vi "SQLDrivers.vi"(4 "error in (no error)":errorcluster, 7 "EnvHandle":i32) -> (0 "error out":errorcluster, 1 "DriverAttributes":string, 2 "DriverDescription":string, 3 "dup EnvHandle":i32)   [LabVIEW 2011]
doc: "Se connecte auprès de la base spécifiée. S'identifie par le nom d'utilisateur et le mot de passe associé"
uses:
  Odbc32.dll
panel:
  out "Overflow 2":i16
  out "Overflow 1":i16
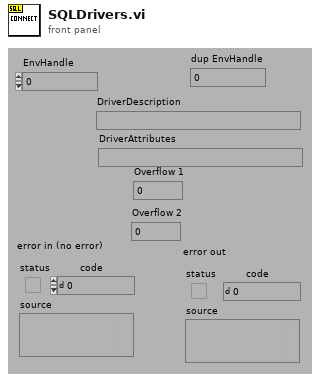
[diagram p1: front panel]
types:
  T1 = enum16{"NOPE", "SQL_HANDLE_ENV", "SQL_HANDLE_DBC", "SQL_HANDLE_STMT", "SQL_HANDLE_DESC"}
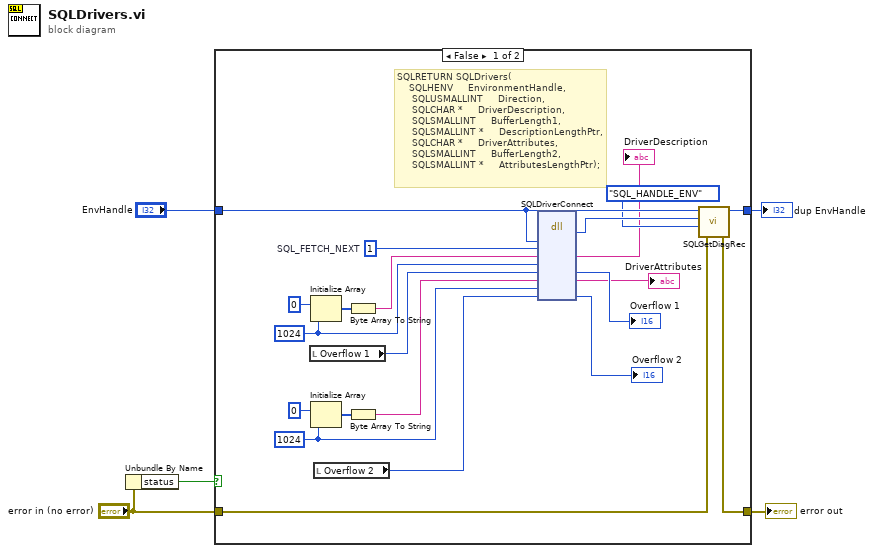
[diagram p0: block diagram]
diagram:
  n1 = Unbundle By Name("error in (no error)") -> ("status"=w4:bool)
  n2 = case shown="False" w4 {
    tunnel: "EnvHandle" -> [w26 w28]
    tunnel: "error in (no error)" -> [w24 w27]
    tunnel: [w23 w27] -> w3
    tunnel: [w25 w28] -> w2
    frame False {
      w9 = i16 1024 ("dimension size")
      w18 = u16 1  # SQL_FETCH_NEXT
      w16 = i16 1024 ("dimension size")
      # "SQLRETURN SQLDrivers(\n    SQLHENV     EnvironmentHandle,\n     SQLUSMALLINT     Direction,\n     SQLCHAR *     DriverDescription,\n     SQLSMALLINT     BufferLength1,\n     SQLSMALLINT *     DescriptionLengthPtr,\n     SQLCHAR *     DriverAttributes,\n     SQLSMALLINT     BufferLength2,\n     SQLSMALLINT *     AttributesLengthPtr);"
      n3 = local read "Overflow 1"() -> (w13:i16)
      n4 = Initialize Array(u8 0, w16) -> (w19:u8[])
      n5 = Initialize Array(u8 0, w9) -> (w12:u8[])
      n6 = local read "Overflow 2"() -> (w8:i16)
      n7 = Byte Array To String(unsigned byte array=w19) -> (string=w17:string)
      n8 = Byte Array To String(unsigned byte array=w12) -> (string=w10:string)
      n9 = dll-call lib="Odbc32.dll" fn="SQLDriverConnect"("EnvironmentHandle"=w26, "Direction"=w18, "DriverDescription"=w17, "BufferLength1"=w16, "DescriptionLengthPtr"=w13, "DriverAttributes"=w10, "BufferLength2"=w9, "AttributesLengthPtr"=w8) -> ("SQLRETURN"=w22:i16, "DriverDescription"=→"DriverDescription":string, "DescriptionLengthPtr"=→"Overflow 1":i16, "DriverAttributes"=→"DriverAttributes":string, "AttributesLengthPtr"=→"Overflow 2":i16)  [unwired: 7 in, 2 out]
      n10 = call "SQLGetDiagRec.vi"("error in (no error)"=w24, "HandleType"=T1."SQL_HANDLE_ENV", "Status (SQL_SUCCESS=0)"=w22, "Input Handle"=w26) -> ("error out"=w23:errorcluster, "Output Handle"=w25:i32)  [unwired: 2 out]
    }
    frame True {
    }
  }
  "dup EnvHandle" <- w2
  "error out" <- w3
